vi "Install Error Codes.vi"() -> ()   [LabVIEW 2021]
panel:
  out "error out":errorcluster
  in  "Custom Error Definition File":string="WebSocket-Actors-errors.txt"
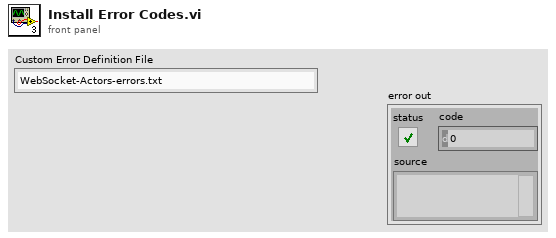
[diagram p1: front panel]
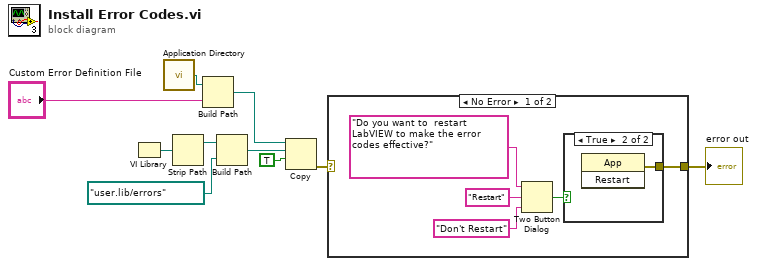
[diagram p0: block diagram]
diagram:
  n1 = VI Library() -> (path=w10:path)
  n2 = call <vilib>:"Application Directory.vi"() -> ("Application Directory"=w7:path)
  n3 = Strip Path(path=w10) -> (stripped path=w8:path)  [unwired: 1 out]
  n4 = Build Path(base path=w7, name or relative path="Custom Error Definition File") -> (appended path=w5:path)
  n5 = Build Path(base path=w8, name or relative path=path "user.lib/errors") -> (appended path=w4:path)
  n6 = Copy(9:TRUE ("overwrite (F)"), 10:w4, 11:w5) -> (0:w2:errorcluster)  [unwired: 2 in, 2 out]
  n7 = case shown="No Error" w2 {
    selector: w2 -> [_ w17]
    tunnel: [w11 w17] -> w1
    frame No Error {
      n8 = Two Button Dialog(message="Do you want to  restart LabVIEW to make the error codes effective?", 1:"Don't Restart" ("F button name (\"Cancel\")"), 2:"Restart" ("T button name (\"OK\")")) -> (T button?=w15:bool)
      n9 = case shown="True" w15 {
        tunnel: [_ w16] -> w11
        frame False {
        }
        frame True {
          n10 = invoke class="App" method="Restart"() -> (error out=w16:errorcluster)  [unwired: 3 in, 2 out]
        }
      }
    }
    frame Error {
    }
  }
  "error out" <- w1
